vi "Do Two Step Build.vi"(8 "error in (no error)":errorcluster, 11 "SDIST in":refnum<class "NI_AB_API_DSDIST.lvclass">) -> (0 "error out":errorcluster, 2 "GeneratedFiles":path[](array[path]), 3 "SDIST out":refnum<class "NI_AB_API_DSDIST.lvclass">)   [LabVIEW 2020, in "NI_AB_API_DSDIST.lvclass"]
uses:
  <vilib>/AppBuilder/AB_API/DSDIST/NI_AB_API_DSDIST.lvclass
  <vilib>/AppBuilder/AB_API/SDIST/NI_AB_API_SDIST.lvclass
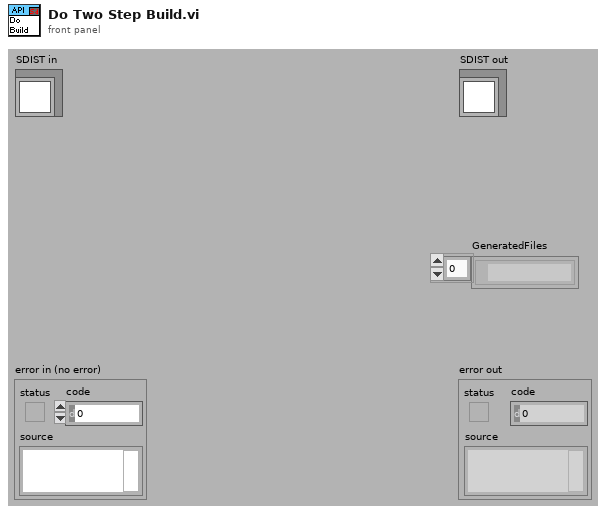
[diagram p1: front panel]
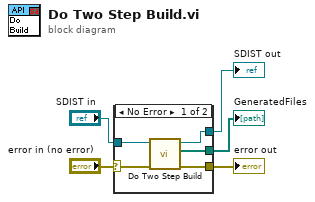
[diagram p0: block diagram]
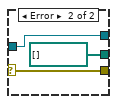
[diagram p2: hidden frame]
diagram:
  n1 = case shown="No Error" "error in (no error)" {
    selector: "error in (no error)" -> [w6 w13]
    tunnel: [w7 w13] -> w4
    tunnel: [w9 w12] -> w2
    tunnel: "SDIST in" -> [w10 w12]
    tunnel: [w8 path[] [] ("GeneratedFiles")] -> w1
    frame No Error {
      n2 = call-parent "Do Two Step Build.vi"("error in (no error)"=w6, "SDIST in"=w10) -> ("error out"=w7:errorcluster, "GeneratedFiles"=w8:path[], "SDIST out"=w9:refnum<class "NI_AB_API_DSDIST.lvclass">)  [unwired: 7 in]
    }
    frame Error {
    }
  }
  "error out" <- w4
  "SDIST out" <- w2
  "GeneratedFiles" <- w1
